vi "Evaluate Script and Read Attribute.vi"(8 "error in (no error)":errorcluster) -> (0 "error out":errorcluster)   [LabVIEW 2020]
uses:
  G-Embedded-Python-Interpreter-Toolkit/Merge Call Library Errors.vi
  <vilib>/addons/_JKI Toolkits/Caraya/classes/Assert/Assert Not Error.vi
  <vilib>/addons/_JKI Toolkits/Caraya/classes/Assert/Assert Error.vi
  <vilib>/addons/_JKI Toolkits/Caraya/classes/Assert/Assert Equal Value_Variant.vi
  G-Embedded-Python-Interpreter-Toolkit/G-Embedded-Python-Interpreter-Toolkit.lvlib
  <vilib>/addons/_JKI Toolkits/Caraya/classes/Assert/Assert.lvclass
  <vilib>/addons/_JKI Toolkits/Caraya/classes/Test/Test.lvclass
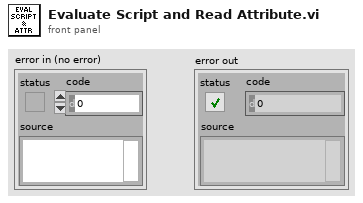
[diagram p1: front panel]
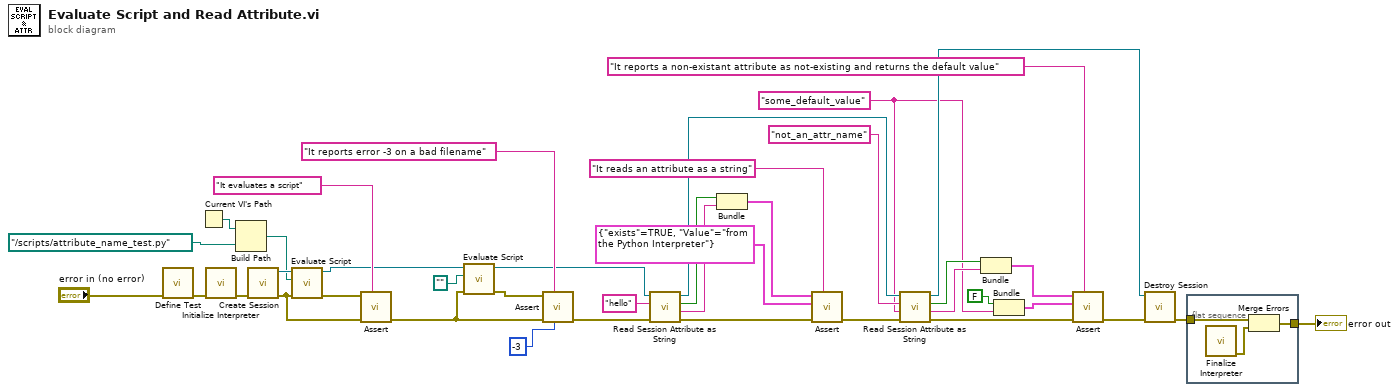
[diagram p0: block diagram]
diagram:
  w9 = "some_default_value" ("Default Value (Empty)")
  n1 = call <vilib>:"Define Test.vi"("error in (no error)"="error in (no error)") -> ("error out"=w40:errorcluster)  [unwired: 10 in]
  n2 = Current VI's Path() -> (path=w35:path)
  n3 = call "Initialize Interpreter.vi"("error in (no error)"=w40) -> ("error out"=w37:errorcluster)  [unwired: 9 in, 1 out]
  n4 = Build Path(base path=w35, name or relative path=path "../scripts/attribute_name_test.py" ("Path")) -> (appended path=w33:path)
  n5 = call "Create Session.vi"("error in (no error)"=w37) -> ("error out"=w31:errorcluster, "Session Handle"=w36:refnum<data-value>)  [unwired: 9 in]
  n6 = call "Evaluate Script.vi"("error in (no error)"=w31, "Script File Path"=w33, "Session Handle in"=w36) -> ("error out"=w32:errorcluster, "Session Handle out"=w29:refnum<data-value>)  [unwired: 7 in]
  n7 = call-poly <vilib>:"Assert.vi"("Label"="It evaluates a script", "error in (no error)"=w31, "Not Error?"=w32) -> ("error out"=w26:errorcluster)  [unwired: 8 in]
  n8 = call "Evaluate Script.vi"("error in (no error)"=w26, "Script File Path"=path "", "Session Handle in"=w29) -> ("error out"=w27:errorcluster, "Session Handle out"=w24:refnum<data-value>)  [unwired: 7 in]
  n9 = call-poly <vilib>:"Assert.vi"("error code (1)"=-3, "Label"="It reports error -3 on a bad filename", "error in (no error)"=w26, "Error?"=w27) -> ("error out"=w23:errorcluster)  [unwired: 7 in]
  n10 = call "Read Session Attribute as String.vi"("error in (no error)"=w23, "Attribute Name"="hello", "Session Handle in"=w24) -> ("error out"=w19:errorcluster, "Value"=w20:string, "Exists"=w21:bool, "Session Handle out"=w16:refnum<data-value>)  [unwired: 5 in]
  n11 = Bundle("Exists"=w21, "Value"=w20) -> (w18:cluster{"Exists":bool, "Value":string})  [unwired: 1 in]
  n12 = call-poly <vilib>:"Assert.vi"("Label"="It reads an attribute as a string", "error in (no error)"=w19, "Y"=cluster{"exists":bool, "Value":string} {"exists"=TRUE, "Value"="from the Python Interpreter"} ("output cluster"), "X"=w18) -> ("error out"=w15:errorcluster)  [unwired: 7 in]
  n13 = call "Read Session Attribute as String.vi"("error in (no error)"=w15, "Default Value (Empty)"=w9, "Attribute Name"="not_an_attr_name", "Session Handle in"=w16) -> ("error out"=w6:errorcluster, "Value"=w11:string, "Exists"=w12:bool, "Session Handle out"=w13:refnum<data-value>)  [unwired: 4 in]
  n14 = Bundle("Exists"=w12, "Value"=w11) -> (w10:cluster{"Exists":bool, "Value":string})  [unwired: 1 in]
  n15 = Bundle(FALSE, "Default Value (Empty)"=w9) -> (w7:cluster{bool, "Default Value (Empty)":string})  [unwired: 1 in]
  n16 = call-poly <vilib>:"Assert.vi"("Label"="It reports a non-existant attribute as not-existing and returns the default value", "error in (no error)"=w6, "Y"=w7, "X"=w10) -> ("error out"=w5:errorcluster)  [unwired: 7 in]
  n17 = call "Destroy Session.vi"("error in (no error)"=w5, "Session Handle"=w13) -> ("error out"=w1:errorcluster)  [unwired: 9 in]
  n18 = flat-sequence {
    tunnel: w1 -> [w43]
    tunnel: [w41] -> w38
    frame #0 {
      n19 = call "Finalize Interpreter.vi"() -> ("error out"=w42:errorcluster)  [unwired: 11 in]
      n20 = Merge Errors(w43, w42) -> (w41:errorcluster)
    }
  }
  "error out" <- w38
